vi "Save File DOE Find Correct Column Location.vi"(8 "error in (no error)":errorcluster, 10 "Search for Header":string[](array[string]), 11 "Calibration With Header":string[][](array[string])=[["Cycle Selection:", "File Paths", "", "Agilent IP", "APLUS IP", "File Search", "", "", "Agilent Channels (Analog)", "Agilent Channels (Temperature TC)", "", "Wash Temperature", "Rinse Temperature", "Load Size", "Model Detail Header", "EOC Commands", "Manufacturer-Dish", "Unit Control-Dish", "Test  Type-Dish", "Cycle Mode-Dish", "Inlet Temperature-Dish", "Detergent-Dish", "Washer Header Detail", "Dishwasher Header Detail", "\"TC1 Coefficients (A_B_C)\"", "\"TC2 Coefficients (A_B_C)\"", "\"TC3 Coefficients (A_B_C)\"", "\"TC4 Coefficients (A_B_C)\"", "\"TC5 Coefficients (A_B_C)\"", "\"TC6 Coefficients (A_B_C)\"", "\"TC7 Coefficients (A_B_C)\"", "TR Number:", "Lab ID:", "Station ID:", "Technician:", "Water Pressure (PSI):", "Ambient RH:", "Supply Voltage:", "Frequency:", "Build:", "Hot Water Temperature (Fahrenheit)", "Cold Water Temperature (Fahrenheit)"], ["Eco Wash", "C:\\GE\\Washer DOE\\CalibrationDates.txt", "", "169.254.9.72", "10.0.3.110", "DOE Template", "", "", "101", "111", "", "Extra Hot", "Cold", "Max", "TR Number:", "EOC", "GE", "Electronic", "Kitchen", "Auto", "110", "Cascade", "Program Name:", "Manufacturer:", "5.00E-05", "4.00E-05", "0", "0", "0", "0", "0", "", "", "Station 1", "", "25", "50", "110", "50", "DG", "120", "50"], ["Standard Wash", "C:\\GE\\Washer DOE\\DOE Capacity.txt", "", "", "", "Rev", "", "", "102", "112", "", "Hot", "Hot Rinse", "Min", "Lab ID:", "ShuttingDown", "Electrolux", "Mechanical", "DOE", "Pots & Pans", "120", "Dawn", "Model Family:", "Unit Control:", "-0.0109", "-0.0092", "0", "0", "0", "0", "0", "", "", "Station 2", "", "30", "60", "115", "60", "DC", "130", "58"], ["Heavy Wash", "C:\\GE\\Washer DOE", "", "", "", "xltm", "", "", "113", "", "", "Warm 1", "", "Avg", "Test Name:", "", "Mabe", "", "", "Quick", "130", "Gain", "Cycle Selection:", "Test Type:", "1.0446", "1.0653", "0", "0", "0", "0", "0", "", "", "Station 3", "", "35", "80", "120", "", "Pre-Pilot", "135", "68"], ["", "\\\\3.67.38.12\\share\\Test Data\\Washer DOE\\Models", "", "", "", "", "", "", "114", "", "", "Warm 2", "", "Max1*", "Model:", "", "Bosch", "", "", "", "135", "", "Wash Temperature:", "Cycle Mode:", "", "", "", "", "", "", "", "", "", "Station 4", "", "", "", "", "", "Production", "140", ""], ["", "D:\\data\\WasherDOE", "", "", "", "", "", "", "115", "", "", "Warm 3", "", "Max2**", "Serial Number:", "", "Whirlpool", "", "", "", "140", "", "Rinse Temperature:", "Inlet Temperature (F):", "", "", "", "", "", "", "", "", "", "Station 5", "", "", "", "", "", "", "", ""], ["", "C:\\GE\\Washer DOE\\DOE_Backup.ini", "", "", "", "", "", "", "116", "", "", "Cold", "", "", "Station ID:", "", "", "", "", "", "", "", "Load Size:", "Detergent:", "", "", "", "", "", "", "", "", "", "Station 6", "", "", "", "", "", "", "", ""], ["", "", "", "", "", "", "", "", "", "", "", "Note ", "", "", "Engineer:", "", "", "", "", "", "", "", "Hot Water Temperature (Fahrenheit):", "Auto Cup Weight (gm):", "", "", "", "", "", "", "", "", "", "Station 7", "", "", "", "", "", "", "", ""], ["", "", "", "", "", "", "", "", "", "", "", "", "", "", "Technician", "", "", "", "", "", "", "", "Cold Water Temperature (Fahrenheit):", "Open Cup Weight (gm):", "", "", "", "", "", "", "", "", "", "Station 8", "", "", "", "", "", "", "", ""], ["", "", "", "", "", "", "", "", "", "", "", "", "", "", "Water Pressure:", "", "", "", "", "", "", "", "Capacity (cu.ft)", "", "", "", "", "", "", "", "", "", "", "Station 9", "", "", "", "", "", "", "", ""], ["", "", "", "", "", "", "", "", "", "", "", "", "", "", "Ambient RH:", "", "", "", "", "", "", "", "Initial Cloth Weight:", "", "", "", "", "", "", "", "", "", "", "Station 10", "", "", "", "", "", "", "", ""], ["", "", "", "", "", "", "", "", "", "", "", "", "", "", "Supply Voltage:", "", "", "", "", "", "", "", "Cloth Lot:", "", "", "", "", "", "", "", "", "", "", "Station 11", "", "", "", "", "", "", "", ""], ["", "", "", "", "", "", "", "", "", "", "", "", "", "", "Frequency:", "", "", "", "", "", "", "", "", "", "", "", "", "", "", "", "", "", "", "Station 12", "", "", "", "", "", "", "", ""], ["", "", "", "", "", "", "", "", "", "", "", "", "", "", "Build:", "", "", "", "", "", "", "", "", "", "", "", "", "", "", "", "", "", "", "", "", "", "", "", "", "", "", ""]]) -> (0 "error out":errorcluster, 3 "Column Index Output":i32)   [LabVIEW 2023, in "File Setup.lvlib"]
uses:
  File Setup.lvlib
  <vilib>/Utility/error.llb/whitespace.ctl
  <vilib>/Utility/error.llb/Trim Whitespace One-Sided.vi
panel:
  # "Search the input header for the correct column number"
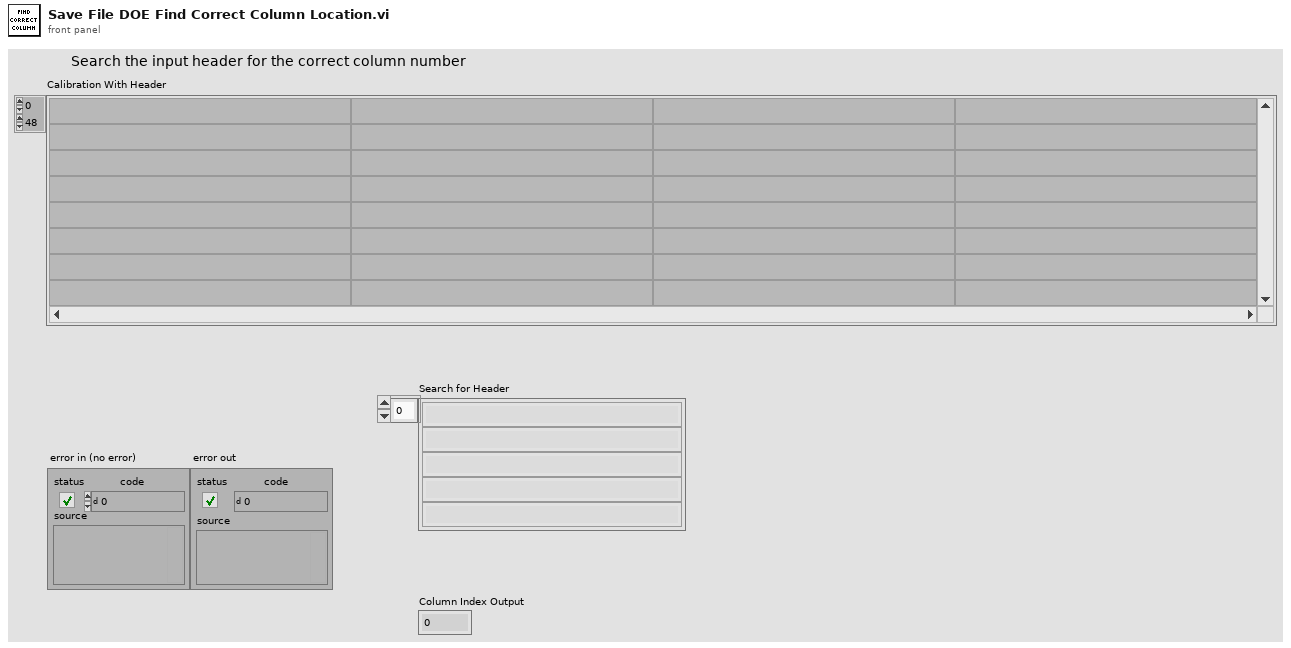
[diagram p1: front panel]
types:
  T1 = typedef "whitespace.ctl" = u16
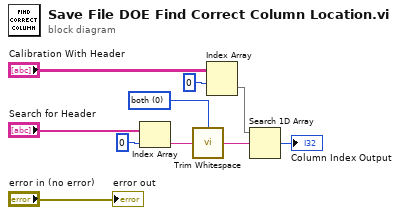
[diagram p0: block diagram]
diagram:
  w1 = T1 0 items=["both", "start of string", "end of string"] ("location (both)")
  n1 = Index Array(array="Search for Header", index=0) -> (element=w3:string)
  n2 = call <vilib>:"Trim Whitespace.vi"("string"=w3, "location (both)"=w1) -> ("trimmed string"=w2:string)
  n3 = Index Array(array="Calibration With Header", index (row)=0) -> (element=w8:string[])  [unwired: 1 in]
  n4 = Search 1D Array(1D array=w8, element=w2) -> (index of element=→"Column Index Output":i32)  [unwired: 1 in]
  "error out" <- "error in (no error)"
